vi "Set Magnet Field.vi"(4 "Axis":T1, 6 "Mode":T2, 8 "error in (no error)":errorcluster, 9 "Target Rate (T/min)":dbl, 10 "Target Field (T)":dbl, 11 "instrument.PPMS2 in":refnum<class "instrument.PPMS2.lvclass">) -> (0 "error out":errorcluster, 3 "instrument.PPMS2 out":refnum<class "instrument.PPMS2.lvclass">)   [LabVIEW 2016, in "instrument.PPMS2.lvclass"]
uses:
  instrument.PPMS2.lvclass
  <userlib>/LevyLab/Levylab Instruments/Instrument Types/Cryostat/Typedefs/Magnet Mode--Enum.ctl
  <userlib>/LevyLab/Levylab Instruments/Instrument Types/Cryostat/Typedefs/Magnet Axis--Enum.ctl
  Typedefs/Magnet Field--PPMS2--cluster.ctl
  <userlib>/LevyLab/Levylab Instruments/Instrument Types/Cryostat/Instrument.Cryostat.lvclass
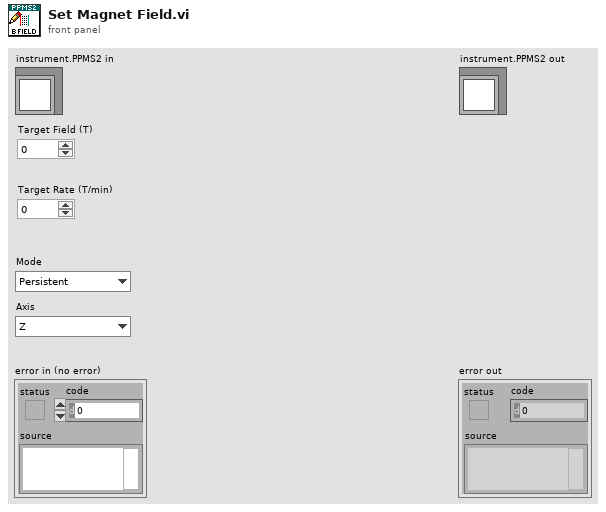
[diagram p1: front panel]
types:
  T1 = typedef "Instrument.Cryostat.lvclass/Magnet Axis--Enum.ctl" = enum16{"Z", "X", "Y"}
  T2 = typedef "Instrument.Cryostat.lvclass/Magnet Mode--Enum.ctl" = enum16{"Persistent", "Driven"}
  T3 = typedef "instrument.PPMS2.lvclass/Magnet Field--PPMS2--cluster.ctl" = cluster{"Target Field (Oe)":dbl, "Target Rate (Oe/s)":dbl, "Mode":T2}
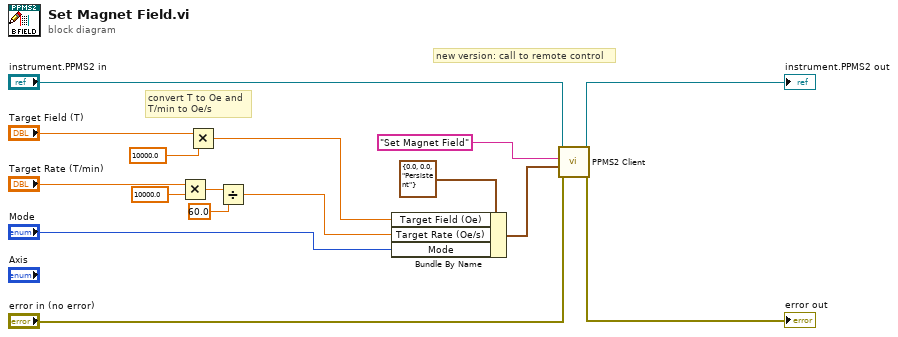
[diagram p0: block diagram]
diagram:
  # "new version: call to remote control"
  # "convert T to Oe and\nT/min to Oe/s"
  n1 = Multiply(x="Target Rate (T/min)", y=10000.0) -> (x*y=w11:dbl)
  n2 = Multiply(x="Target Field (T)", y=10000.0) -> (x*y=w6:dbl)
  n3 = Divide(x=w11, y=60.0) -> (x/y=w5:dbl)
  n4 = Bundle By Name(cluster=T3 {"Target Field (Oe)"=0.0, "Target Rate (Oe/s)"=0.0, "Mode"=enum."Persistent"} ("output cluster"), "Target Field (Oe)"=w6, "Target Rate (Oe/s)"=w5, "Mode"="Mode") -> (w1:T3)
  n5 = call "PPMS2 Client.vi"("error in (no error)"="error in (no error)", "Data"=w1, "Command"="Set Magnet Field", "instrument.PPMS2 in"="instrument.PPMS2 in") -> ("error out"=→"error out":errorcluster, "instrument.PPMS2 out"=→"instrument.PPMS2 out":refnum<class "instrument.PPMS2.lvclass">)  [unwired: 4 in, 2 out]
